vi "Operator message space bar continue with bool dont do.vi"(8 "error in (no error)":errorcluster, 9 "Dont do?":bool, 10 "Message.Font:Size":u32=36, 11 "Message":string) -> (0 "error out":errorcluster, 3 "Time waiting in secs":string)   [LabVIEW 2013]
uses:
  <vilib>/event_ctls.llb/eventvkey.ctl
panel:
  # "Operator Message"
  # "Press SPACE BAR to continue"
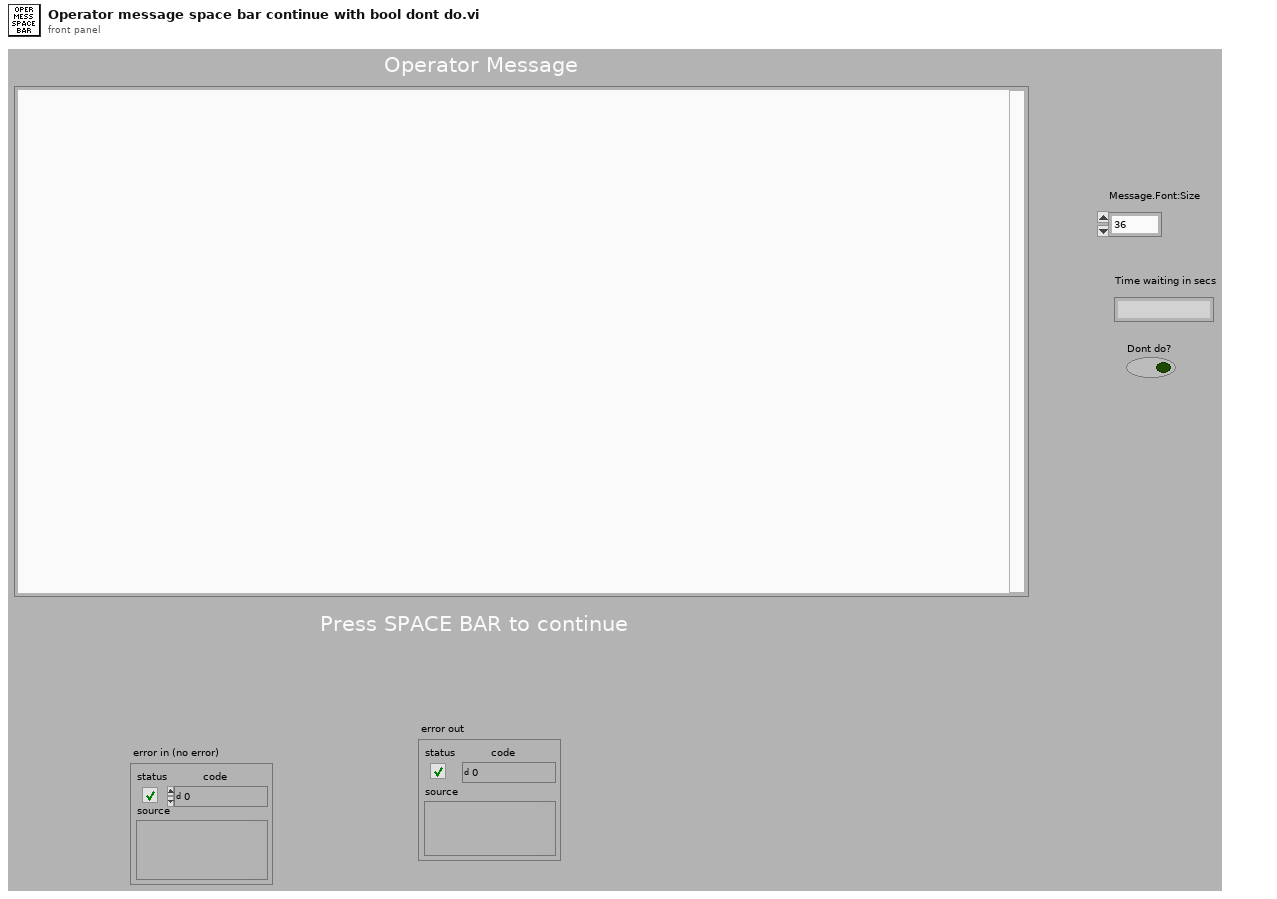
[diagram p1: front panel]
types:
  T1 = typedef "eventvkey.ctl" = enum16{"ASCII", "Enter", "Return", "Shift", "Ctrl", "Alt", "Cmd", "Opt", "Caps", "NumLock", "Clear", "Break", "Up", "Down", "Left", "Right", "Insert", "Delete", "Home", "End", "PageUp", "PageDown", "Escape", "Help", "Pause", "ScrollLock", "F1", "F2", "F3", "F4", "F5", "F6", "F7", "F8", "F9", "F10", "F11", "F12", "F13", "F14", "F15", "F16", "F17", "F18", "F19", "F20", "F21", "F22", "F23", "F24", "Play", "VolumeUp", "VolumeDown", "Mute", "Two Byte Char"}
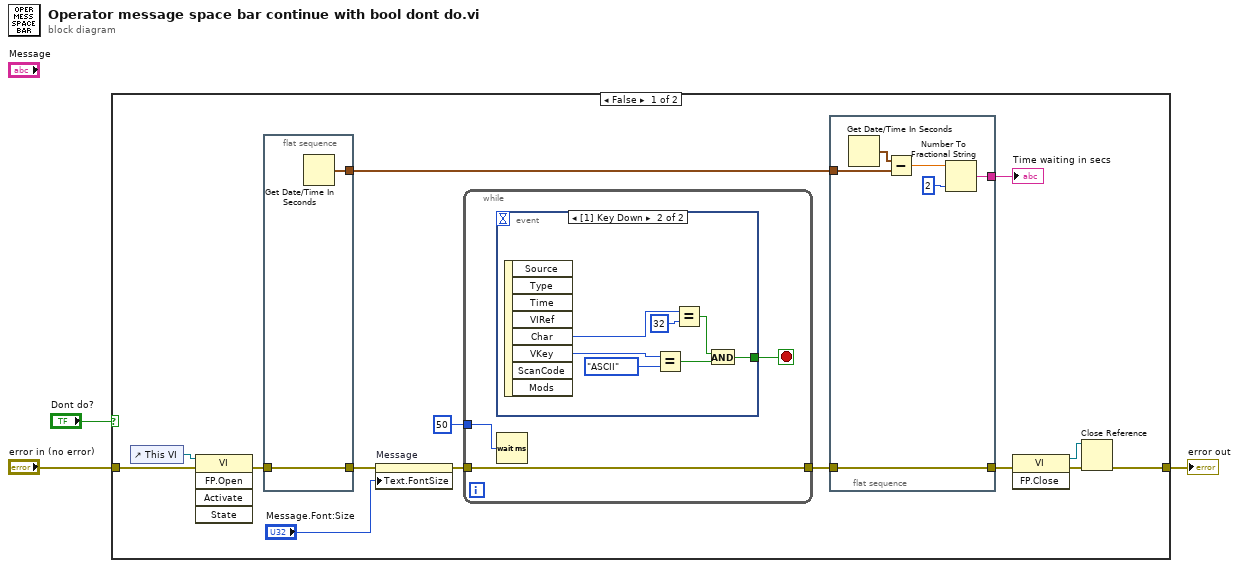
[diagram p0: block diagram]
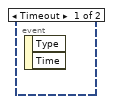
[diagram p2: hidden frame]
diagram:
  n1 = case shown="False" "Dont do?" {
    tunnel: "error in (no error)" -> [w9 w36]
    tunnel: [w4 w36] -> w2
    frame False {
      n2 = control-ref of="This VI"() -> (w10:refnum<vi>)
      n3 = invoke class="VI" method="FP.Open"(reference=w10, error in=w9) -> (error out=w8:errorcluster)  [unwired: 3 in, 4 out]
      n4 = flat-sequence {
        tunnel: [w25] -> w14
        tunnel: w8 -> [w25]
        tunnel: [w24] -> w12
        frame #0 {
          n5 = Get Date/Time In Seconds() -> (seconds since 1Jan1904=w24:timestamp)
        }
      }
      n6 = property on="Message" class="Str"(error in=w14, "Text.FontSize"="Message.Font:Size") -> (error out=w16:errorcluster)  [unwired: 1 in, 1 out]
      n7 = while {
        tunnel: u32 50 ("milliseconds to wait") -> [w28]
        tunnel: [w26] -> w13
        tunnel: w16 -> [w26]
        stop <- w27 stop-if-true
        n8 = event shown="[1] Key Down" {
          selector: _ -> [_ _]
          dyn-events: _ -> [_ _]
          timeout: _ -> [_ _]
          tunnel: [_ w29] -> w27
          event Timeout {
            n9 = event-data() -> ()  [unwired: 1 in, 2 out]
          }
          event Key Down {
            n10 = event-data() -> ("Char"=w35:i16, "VKey"=w33:T1)  [unwired: 1 in, 6 out]
            n11 = Equal?(x=w33, y=eventvkey."ASCII" ("VKey")) -> (x = y?=w30:bool)
            n12 = Equal?(x=w35, y=i16 32) -> (x = y?=w31:bool)
            n13 = And(x=w31, y=w30) -> (x .and. y?=w29:bool)
          }
        }
        n14 = Wait (ms)(milliseconds to wait=w28) -> ()  [unwired: 1 out]
      }
      n15 = flat-sequence {
        tunnel: [w23] -> w7
        tunnel: w13 -> [w23]
        tunnel: w12 -> [w21]
        tunnel: [w18] -> w11
        frame #0 {
          n16 = Get Date/Time In Seconds() -> (seconds since 1Jan1904=w22:timestamp)
          n17 = Subtract(x=w22, y=w21) -> (x-y=w20:dbl)
          n18 = Number To Fractional String(number=w20, precision (6)=i16 2) -> (F-format string=w18:string)  [unwired: 2 in]
        }
      }
      n19 = invoke class="VI" method="FP.Close"(error in=w7) -> (reference out=w6:refnum<vi>, error out=w5:errorcluster)  [unwired: 2 in, 1 out]
      n20 = Close Reference(reference=w6, error in (no error)=w5) -> (error out=w4:errorcluster)
      "Time waiting in secs" <- w11
    }
    frame True {
    }
  }
  "error out" <- w2
